vi "Dashboard Main.vi"() -> ()   [LabVIEW 2019]
uses:
  <vilib>/Rock Robotics/Network Tables/NT Read Numeric Array.vi
  <vilib>/Rock Robotics/Network Tables/NT Read Number.vi
  <vilib>/Rock Robotics/Network Tables/NT Read Boolean.vi
  <vilib>/Rock Robotics/Network Tables/NT Read String.vi
  <vilib>/Rock Robotics/Network Tables/NT Read Boolean Array.vi
  <vilib>/Rock Robotics/WPI/ThirdParty/JAS_Junk/TrajLib/Trajectory_Library.lvlib
panel:
  out "Camera Perf":string
  in  "Camera Settings":T1={"Frame Rate"=30, "Compression"=30, "Size"=1, "DB Camera Config"=FALSE} {"Frame Rate" scale=1.0..30.0; "Compression" scale=100.0..-1.0; "Size" items=["640x480", "320x240", "160x120"]}
  in  "TCP":refnum<k5>
  out "Robot IP":string
  in  "Dashboard Tab":T2(tab)
  out "MotorChart R":cluster{"Numeric":dbl, "Numeric":dbl}(graph)
  out "MotorChart L":cluster{"Numeric":dbl, "Numeric":dbl}(graph)
  out "MotorSliders R":cluster{"MotorSlide1":dbl, "MotorSlide2":dbl} {"MotorSlide2" scale=-1.0..1.0 scale format="%#_2e"; "MotorSlide1" scale=-1.0..1.0 scale format="%#_2e"}
  out "MotorSliders L":cluster{"MotorSlide1":dbl, "MotorSlide2":dbl} {"MotorSlide2" scale=-1.0..1.0 scale format="%#_2e"; "MotorSlide1" scale=-1.0..1.0 scale format="%#_2e"}
  out "JS1 Z":dbl(slide) scale=-1.0..1.0 scale format="%#_2e"
  out "JS1 Graph":cluster{"X":dbl, "Y":dbl}[](graph)
  out "JS1 Buttons":T3
  out "JS2 Z":dbl(slide) scale=-1.0..1.0 scale format="%#_2e"
  out "JS2 Graph":cluster{"X":dbl, "Y":dbl}[](graph)
  out "JS2 Buttons":T3
  out "Mode":T4(ring)=enum."Auto Disabled"
  in  "DB/String 9":string
  in  "DB/String 8":string
  in  "DB/String 7":string
  in  "DB/String 6":string
  in  "DB/String 5":string
  in  "DB/String 4":string
  in  "DB/String 3":string
  in  "DB/String 2":string
  in  "DB/String 1":string
  in  "DB/String 0":string
  in  "DB/Slider 0":dbl(slide) scale=0.0..5.0
  in  "DB/Slider 1":dbl(slide) scale=0.0..5.0
  in  "DB/Slider 2":dbl(slide) scale=0.0..5.0
  in  "DB/Slider 3":dbl(slide) scale=0.0..5.0
  out "DB/LED 3":bool
  out "DB/LED 2":bool
  out "DB/LED 1":bool
  out "DB/LED 0":bool
  in  "DB/Button 3":bool
  in  "DB/Button 2":bool
  in  "DB/Button 1":bool
  in  "DB/Button 0":bool caption="New Name"
  out "Gyro":dbl format="%10.1f"
  out "Gauge 2":dbl(knob) scale=-180.0..180.0
  out "Auto":bool
  out "R Err":dbl format="%9.2f"
  out "R Speed":dbl format="%10.1f"
  out "R Dmd":dbl format="%10.1f"
  out "L Err":dbl format="%9.2f"
  out "L Speed":dbl format="%10.1f"
  out "L Dmd":dbl format="%10.1f"
  out "NT Connection":bool
  in  "Select Auto":string(combo)="Select Autonomous ..."
  out "At Reference -":bool
  out "Ramsete Enabled -":bool
  out "Left Kp":dbl format="%13.3f"
  out "Left Ki":dbl format="%13.3f"
  out "Right Kp":dbl format="%13.3f"
  out "Right Ki":dbl format="%13.3f"
  out "Auto Tune Engaged":bool
  in  "Start Drive\nSpin Auto Tune":bool
  out "AutoTune\nRight Error":bool
  out "AutoTune\nLeft Error":bool
  out "AutoTune\nRight Done":bool
  out "AutoTune\nLeft Done":bool
  out "Test Name":string
  out "Test Step":string
  out "Test Step Time":dbl format="%16.1f"
  out "Left CO Offset":dbl format="%13.3f"
  out "Right CO Offset":dbl format="%13.3f"
  in  "Start Drive\nFwd Auto Tune":bool
  out "Drive Left":T5(graph)
  out "Drive Right":T5(graph)
  out "Ramsete Enabled":bool
  out "At Reference":bool
  out "Traj Error":T5(graph)
  out "Tree":string(tree)
  out "Camera Image":T6(plugin-control)
  out "Background":bool
  in  "Camera Name":string(combo)="No Camera Selection"
  # "HW"
  # "Joysticks"
  # "Drive Motors"
  # "Front"
  # "Right"
  # "Left"
  # "Back"
  # "Drive"
  # "Trajectory"
  # "Feet, Feet, Degrees/10"
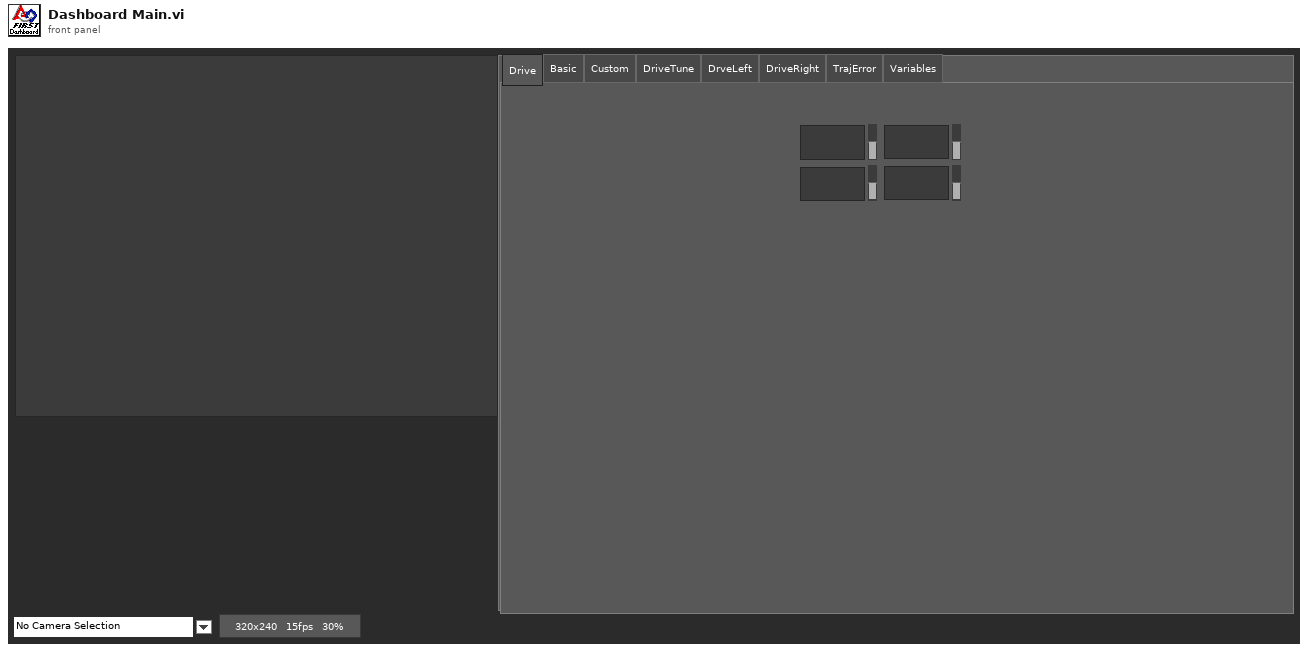
[diagram p1: front panel]
types:
  T1 = cluster{"Frame Rate":i32, "Compression":i32, "Size":u16, "DB Camera Config":bool}
  T2 = enum32{"Drive", "Basic", "Custom", "DriveTune", "DrveLeft", "DriveRight", "TrajError", "Variables"}
  T3 = cluster{bool, bool, bool, bool, bool, bool, bool, bool, bool, bool, bool, bool}
  T4 = enum8{"Tele-Op Disabled", "Tele-Op Enabled", "Auto Disabled", "Auto Enabled", "Test Disabled", "Test Enabled", "Disconnected", "No Code", "E-Stop"}
  T5 = cluster{"Numeric":dbl, "Numeric":dbl, "Numeric":dbl}
  T6 = typedef "IMAQ Image.ctl" = refnum<image>
  T7 = cluster{"Save Path":path, "Interval (s)":dbl, "Keep":i32}
  T8 = typedef "Image Type" = u32
  T9 = cluster{"Camera Image":refnum<vi>, "Dashboard Tab":refnum<vi>, "Background":refnum<vi>, "Tree":refnum<vi>, "Camera Settings":refnum<vi>, "Camera Name":refnum<vi>, "Camera Perf":refnum<vi>}
  T10 = cluster{"Shift":bool, "Ctrl":bool, "Alt":bool, "Cmd":bool, "Opt":bool}
  T11 = cluster{"Error Strings":string, "Disable Counts":cluster{u16, u16}, "Rail Faults":cluster{u16, u16, u16}, "Robot IP":string, "DB Mode":u8, "Event Info":cluster{"Name":string, "Type":u8, "Number":u16, "Replay":u8}}
  T12 = cluster{"Storage":cluster{"Disk Free":u64, "RAM Block":u32, "RAM free":u32}, "CPU Utilization":cluster{"CPU % ISR":sgl, "CPU % Time Crit":sgl, "CPU % Timed Str":sgl, "CPU % High":sgl, "CPU % Above":sgl, "CPU % Normal":sgl, "CPU % Low":sgl}, "CAN":cluster{"% Bus Utilization":sgl, "Bus Off Cnt":u32, "TX_FIFO Full Cnt":u32, "Receive Error Cnt":u8, "Transmit Error Cnt":u8}, "HID":cluster{"HID Outputs":u32, "Rumble Low":u16, "Rumble High":u16}[]}
  T13 = cluster{"Status bits":cluster{"Test Mode":bool, "Autonomous":bool, "Enabled":bool, "Code Start":bool, "Brownout":bool, "Reserved 2":bool, "Reserved 3":bool, "E-Stop":bool}, "Code Trace":cluster{"Disabled":bool, "TeleOp":bool, "Auto":bool, "Test":bool}, "Controller Type":enum16{"unknown", "cRIO", "roboRio"}, "Code?":enum16{"unknown", "noCode", "code"}, "Battery V":dbl}
  T14 = cluster{"Control Bits":cluster{"TestMode":bool, "Autonomous":bool, "Enabled":bool, "FMS Present":bool, bool, bool, bool, "E-Stop":bool}, "Team Station ":u8, "Countdown":sgl, "Joystick Values":cluster{"Axes":dbl[], "Buttons":bool[], "POVs":i16[]}[]}
  T15 = cluster{"Axes":dbl[], "Buttons":bool[], "POVs":i16[]}[]
  T16 = cluster{"Axes":dbl[], "Buttons":bool[], "POVs":i16[]}
  T17 = cluster{"Buttons[0]":bool, "Buttons[1]":bool, "Buttons[2]":bool, "Buttons[3]":bool, "Buttons[4]":bool, "Buttons[5]":bool, "Buttons[6]":bool, "Buttons[7]":bool, "Buttons[8]":bool, "Buttons[9]":bool, "Buttons[10]":bool, "Buttons[11]":bool}
  T18 = cluster{"Camera Name":string, "Camera File Name":string, "Saved DB Images Info":cluster{"Save Path":path, "Interval (s)":dbl, "Keep":i32}}
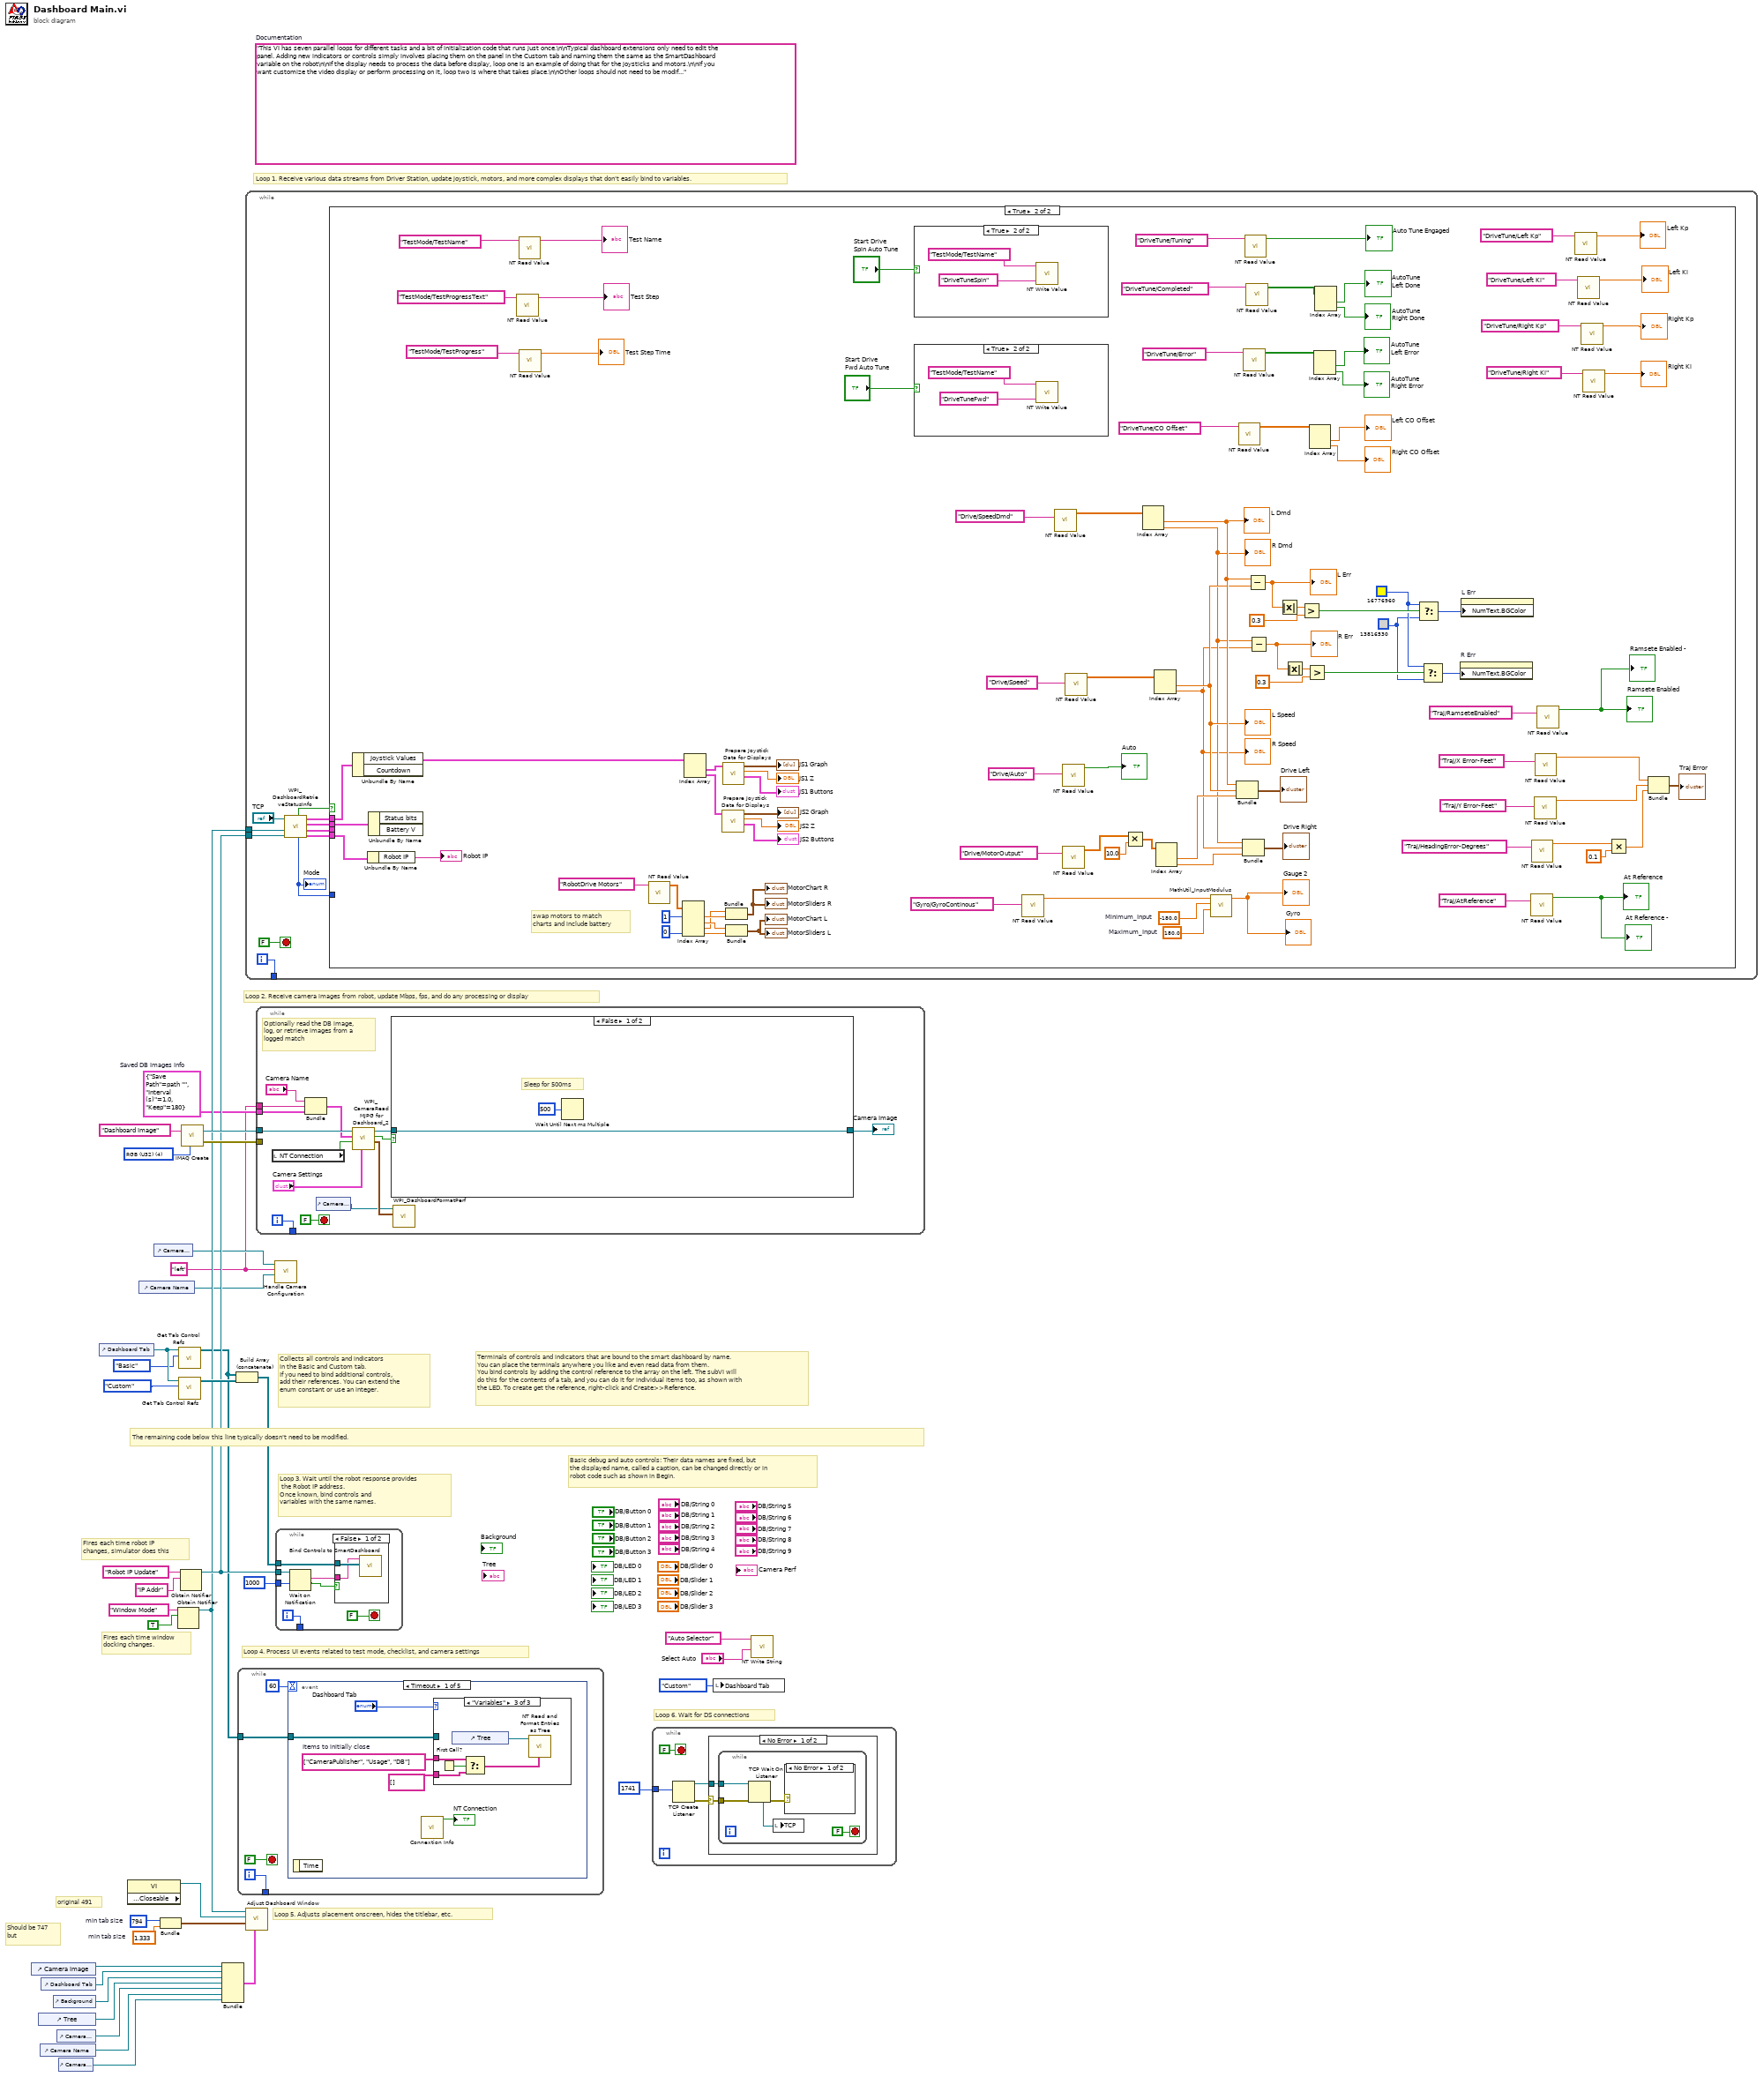
[diagram p0: block diagram]
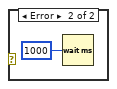
[diagram p2: hidden frame]
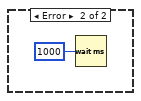
[diagram p3: hidden frame]
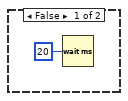
[diagram p4: hidden frame]
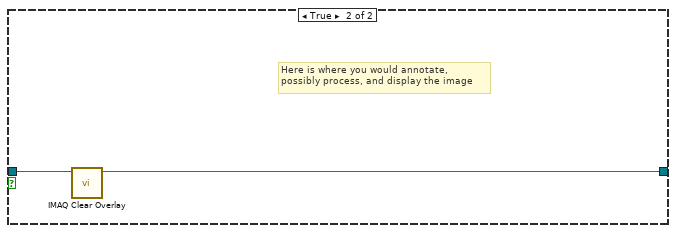
[diagram p8: hidden frame]
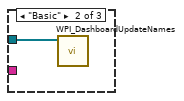
[diagram p10: hidden frame]
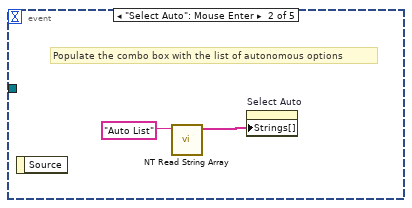
[diagram p11: hidden frame]
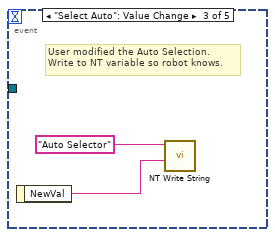
[diagram p12: hidden frame]
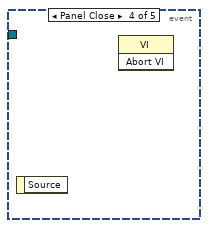
[diagram p13: hidden frame]
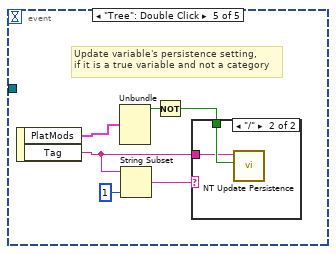
[diagram p14: hidden frame]
diagram:
  w2 = "left" ("Camera File Name")
  w3 = T7 {"Save Path"=path "", "Interval (s)"=1.0, "Keep"=180}  # Saved DB Images Info
  w22 = 794  # min tab size
  w21 = 1.333  # min tab size
  (unwired) "This VI has seven parallel loops for different tasks and a bit of initialization code that runs just once.\n\nTypical dashboard extensions only need to edit the panel. Adding new indicators or controls simply involves placing them on the panel in the Custom tab and naming them the same as the SmartDashboard variable on the robot\n\nIf the display needs to process the data before display, loop one is an example of doing that for the joysticks and motors.\n\nIf you want customize the video display or perform processing on it, loop two is where that takes place.\n\nOther loops should not need to be modified. They are pretty standard, and document the task they perform."  # Documentation
  w37 = T8 4 items=["Grayscale (U8)", "Grayscale (I16)", "Grayscale (SGL)", "Complex (CSG)", "RGB (U32)", "HSL (U32)", "RGB (U64)"] ("Image Type")
  # "Should be 747\nbut"
  # "original 491"
  # "Loop 6. Wait for DS connections"
  # "Basic debug and auto controls: Their data names are fixed, but\nthe displayed name, called a caption, can be changed directly or in\nrobot code such as shown in Begin."
  # "Fires each time robot IP\nchanges, simulator does this"
  # "Fires each time window\ndocking changes."
  # "Collects all controls and indicators\nin the Basic and Custom tab.\nIf you need to bind additional controls,\nadd their references. You can extend the\nenum constant or use an integer."
  # "The remaining code below this line typically doesn't need to be modified."
  # "Loop 4. Process UI events related to test mode, checklist, and camera settings"
  # "Terminals of controls and indicators that are bound to the smart dashboard by name.\nYou can place the terminals anywhere you like and even read data from them.\nYou bind controls by adding the control reference to the array on the left. The subVI will\ndo this for the contents of a tab, and you can do it for individual items too, as shown with\nthe LED. To create get the reference, right-click and Create>>Reference."
  # "Loop 3. Wait until the robot response provides\n the Robot IP address.\nOnce known, bind controls and\nvariables with the same names."
  # "Loop 5. Adjusts placement onscreen, hides the titlebar, etc."
  # "Loop 1. Receive various data streams from Driver Station, update joystick, motors, and more complex displays that don't easily bind to variables."
  # "Loop 2. Receive camera images from robot, update Mbps, fps, and do any processing or display"
  n1 = control-ref of="Camera Image"() -> (w24:refnum<vi>)
  n2 = control-ref of="Tree"() -> (w9:refnum<vi>)
  n3 = control-ref of="Camera Name"() -> (w7:refnum<vi>)
  n4 = control-ref of="Dashboard Tab"() -> (w23:refnum<vi>)
  n5 = control-ref of="Background"() -> (w19:refnum<vi>)
  n6 = control-ref of="Camera Settings"() -> (w8:refnum<vi>)
  n7 = control-ref of="Camera Perf"() -> (w6:refnum<vi>)
  n8 = control-ref of="Dashboard Tab"() -> (w27:refnum<vi>)
  n9 = property class="VI" props=["Front Panel.Closeable"]() -> (reference out=w28:refnum<vi>)  [unwired: 2 in, 2 out]
  n10 = control-ref of="Camera Name"() -> (w13:refnum<vi>)
  n11 = control-ref of="Camera Settings"() -> (w14:refnum<vi>)
  n12 = Bundle("min tab size"=w22, "min tab size"=w21) -> (w20:cluster{"min tab size":i32, "min tab size":dbl})  [unwired: 1 in]
  n13 = Obtain Notifier(name (unnamed)="Window Mode", notification data type=TRUE) -> (notifier out=w16:refnum<notifier>)  [unwired: 2 in, 2 out]
  n14 = call <vilib>:"Get Tab Control Refs.vi"("Page Index"=enum32{"Drive", "Basic", "Custom", "Variables"}."Basic" ("Dashboard Tab"), "TabControl in"=w27) -> ("ControlsOnPage"=w12:refnum<vi>[])  [unwired: 9 in]
  n15 = call <vilib>:"Get Tab Control Refs.vi"("Page Index"=enum32{"Drive", "Basic", "Custom", "Variables"}."Custom" ("Dashboard Tab"), "TabControl in"=w27) -> ("ControlsOnPage"=w26:refnum<vi>[])  [unwired: 9 in]
  n16 = Obtain Notifier(name (unnamed)="Robot IP Update", notification data type="IP Addr" ("name (unnamed)")) -> (notifier out=w17:refnum<notifier>)  [unwired: 2 in, 2 out]
  n17 = call "IMAQ Create"("Image Name"="Dashboard Image", "Image Type"=w37) -> ("New Image"=w35:T6, "error out"=w34:errorcluster)  [unwired: 2 in, 1 out]
  n18 = Bundle("Camera Image"=w24, "Dashboard Tab"=w23, "Background"=w19, "Tree"=w9, "Camera Settings"=w8, "Camera Name"=w7, "Camera Perf"=w6) -> (w18:T9)  [unwired: 1 in]
  n19 = Build Array (concatenate)(w12, w26) -> (w25:refnum<vi>[])
  n20 = while {
    tunnel: [w39] -> _
    tunnel: w12 -> [w38]
    i -> [w39]
    stop <- FALSE stop-if-true
    n21 = event shown="[0] Timeout" {
      selector: _ -> [_ _ _ _ _]
      dyn-events: _ -> [_ _ _ _ _]
      timeout: u32 60 ("milliseconds to wait") -> [_ _ _ _ _]
      tunnel: w38 -> [w44 _ _ _ _]
      event Timeout {
        w43 = string[] ["CameraPublisher", "Usage", "DB"]  # Items to initially close
        n22 = event-data() -> ()  [unwired: 1 in, 1 out]
        n23 = call <vilib>:"Connextion Info.vi"() -> ("Connected"=→"NT Connection":bool)  [unwired: 10 in, 1 out]
        n24 = case shown="\"Variables\"" "Dashboard Tab" {
          tunnel: w44 -> [_ w47 _]
          tunnel: w43 -> [_ _ w50]
          tunnel: string[] [] -> [_ _ w49]
          frame "Custom", Default {
          }
          frame "Basic" {
            n25 = call <vilib>:"WPI_DashboardUpdateNames.vi"("Controls on Tab"=w47) -> ()  [unwired: 11 in]
          }
          frame "Variables" {
            n26 = First Call?() -> (First Call?: T/F=w51:bool)
            n27 = control-ref of="Tree"() -> (w52:refnum<vi>)
            n28 = Select(t=w50, s=w51, f=w49) -> (s? t:f=w48:string[])
            n29 = call <vilib>:"NT Read and Format Entries as Tree.vi"("Tags to  Close"=w48, "Tree Refnum"=w52) -> ()  [unwired: 8 in, 2 out]
          }
        }
      }
      event "Select Auto": Mouse Enter {
        # "Populate the combo box with the list of autonomous options"
        n30 = event-data() -> ()  [unwired: 1 in, 1 out]
        n31 = call <vilib>:"NT Read String Array.vi"("Name"="Auto List") -> ("String Array"=w53:string[])  [unwired: 9 in, 1 out]
        n32 = property on="Select Auto" class="CmbBox"("Strings[]"=w53) -> ()  [unwired: 2 in, 2 out]
      }
      event "Select Auto": Value Change {
        # "User modified the Auto Selection.\nWrite to NT variable so robot knows."
        n33 = event-data() -> ("NewVal"=w55:string)  [unwired: 1 in]
        n34 = call <vilib>:"NT Write String.vi"("String"=w55, "Name"="Auto Selector") -> ()  [unwired: 9 in, 1 out]
      }
      event Panel Close {
        n35 = event-data() -> ()  [unwired: 1 in, 1 out]
        n36 = invoke class="VI" method="Abort VI"() -> ()  [unwired: 3 in, 3 out]
      }
      event "Tree": Double Click {
        # "Update variable's persistence setting,\nif it is a true variable and not a category"
        n37 = event-data() -> ("PlatMods"=w58:T10, "Tag"=w57:string)  [unwired: 1 in]
        n38 = Unbundle(w58) -> ("Shift"=w62:bool)  [unwired: 4 out]
        n39 = String Subset(string=w57, length (rest)=1 ("length (rest)")) -> (substring=w59:string)  [unwired: 1 in]
        n40 = Not(x=w62) -> (.not. x?=w61:bool)
        n41 = case shown="\"/\"" w59 {
          tunnel: w61 -> [_ w64]
          tunnel: w57 -> [_ w63]
          frame Default {
          }
          frame "/" {
            n42 = call <vilib>:"NT Update Persistence.vi"("Persistence"=w64, "Name"=w63) -> ()  [unwired: 9 in, 1 out]
          }
        }
      }
    }
  }
  n43 = while {
    tunnel: [w74] -> _
    tunnel: w17 -> [w68]
    tunnel: w16 -> [w65]
    i -> [w74]
    stop <- FALSE stop-if-true
    n44 = call <vilib>:"WPI_DashboardRetrieveStatusInfo.vi"("Binding Refnum"=w68, "Window Mode Notifier"=w65, "TCP Cnx"="TCP") -> ("Power and Errors"=w69:T11, "Robot Metrics"=w72:T12, "Status Info"=w73:T13, "Control Info"=w70:T14, "Robot Mode"=w67:T4, "Process?"=w71:bool)  [unwired: 3 in]
    "Mode" <- w67
    n45 = case shown="True" w71 {
      tunnel: w73 -> [_ w177]
      tunnel: w72 -> [_ _]
      tunnel: w70 -> [_ w176]
      tunnel: w69 -> [_ w175]
      tunnel: w67 -> [_ _]
      frame False {
        n46 = Wait (ms)(milliseconds to wait=u32 20) -> ()  [unwired: 1 out]
      }
      frame True {
        w115 = -180.0  # Minimum_Input
        w114 = 180.0  # Maximum_Input
        w119 = u32 13816530
        w120 = u32 16776960
        # "swap motors to match\ncharts and include battery"
        n47 = Unbundle By Name(w176) -> ("Joystick Values"=w166:T15)  [unwired: 1 out]
        n48 = Unbundle By Name(w175) -> ("Robot IP"=→"Robot IP":string)
        n49 = Unbundle By Name(w177) -> ()  [unwired: 2 out]
        n50 = call-poly <vilib>:"NT Read Value.vi"("Name"="TestMode/TestProgressText") -> ("String"=→"Test Step":string)  [unwired: 9 in, 1 out]
        n51 = call-poly <vilib>:"NT Read Value.vi"("Name"="TestMode/TestName") -> ("String"=→"Test Name":string)  [unwired: 9 in, 1 out]
        n52 = call-poly <vilib>:"NT Read Value.vi"("Name"="TestMode/TestProgress") -> ("Numeric"=→"Test Step Time":dbl)  [unwired: 9 in, 1 out]
        n53 = call-poly <vilib>:"NT Read Value.vi"("Name"="RobotDrive Motors") -> ("Numeric Array"=w156:dbl[])  [unwired: 9 in, 1 out]
        n54 = Index Array(array=w156, index #1=1, index #4=0) -> (element #1=w170:dbl, element #2=w171:dbl, element #3=w169:dbl, element #4=w174:dbl)  [unwired: 2 in]
        n55 = Index Array(array=w166) -> (element #1=w165:T16, element #2=w161:T16)  [unwired: 2 in]
        n56 = call "Prepare Joystick Data for Displays.vi"("Joystick Values"=w161) -> ("Buttons"=→"JS2 Buttons":T17, "Z Axis"=→"JS2 Z":dbl, "Cartesian Data"=→"JS2 Graph":cluster{"X axis":dbl, "X axis":dbl}[])  [unwired: 8 in]
        n57 = call "Prepare Joystick Data for Displays.vi"("Joystick Values"=w165) -> ("Buttons"=→"JS1 Buttons":T17, "Z Axis"=→"JS1 Z":dbl, "Cartesian Data"=→"JS1 Graph":cluster{"X axis":dbl, "X axis":dbl}[])  [unwired: 8 in]
        n58 = Bundle("Numeric"=w169, "Numeric"=w170) -> (→"MotorChart R" →"MotorSliders R":cluster{"Numeric":dbl, "Numeric":dbl})  [unwired: 1 in]
        n59 = Bundle("Numeric"=w171, "Numeric"=w174) -> (→"MotorChart L" →"MotorSliders L":cluster{"Numeric":dbl, "Numeric":dbl})  [unwired: 1 in]
        n60 = case shown="True" "Start Drive\nSpin Auto Tune" {
          frame False {
          }
          frame True {
            n61 = call-poly <vilib>:"NT Write Value.vi"("String"="DriveTuneSpin", "Name"="TestMode/TestName") -> ()  [unwired: 9 in, 1 out]
          }
        }
        n62 = case shown="True" "Start Drive\nFwd Auto Tune" {
          frame False {
          }
          frame True {
            n63 = call-poly <vilib>:"NT Write Value.vi"("String"="DriveTuneFwd", "Name"="TestMode/TestName") -> ()  [unwired: 9 in, 1 out]
          }
        }
        n64 = call-poly <vilib>:"NT Read Value.vi"("Name"="Gyro/GyroContinous") -> ("Numeric"=w113:dbl)  [unwired: 9 in, 1 out]
        n65 = call-poly <vilib>:"NT Read Value.vi"("Name"="Drive/SpeedDmd") -> ("Numeric Array"=w151:dbl[])  [unwired: 9 in, 1 out]
        n66 = call-poly <vilib>:"NT Read Value.vi"("Name"="Drive/Auto") -> ("Boolean"=→"Auto":bool)  [unwired: 9 in, 1 out]
        n67 = call-poly <vilib>:"NT Read Value.vi"("Name"="Drive/MotorOutput") -> ("Numeric Array"=w109:dbl[])  [unwired: 9 in, 1 out]
        n68 = call-poly <vilib>:"NT Read Value.vi"("Name"="Drive/Speed") -> ("Numeric Array"=w150:dbl[])  [unwired: 9 in, 1 out]
        n69 = Multiply(x=w109, y=10.0) -> (x*y=w108:dbl[])
        n70 = Index Array(array=w151) -> (element #1=w134:dbl, element #2=w132:dbl)  [unwired: 2 in]
        "L Dmd" <- w134
        "R Dmd" <- w132
        n71 = Index Array(array=w150) -> (element #1=w133:dbl, element #2=w131:dbl)  [unwired: 2 in]
        "L Speed" <- w133
        "R Speed" <- w131
        n72 = Index Array(array=w108) -> (element #1=w149:dbl, element #2=w148:dbl)  [unwired: 2 in]
        n73 = call <vilib>:"MathUtil_InputModulus.vi"("Maximum_Input"=w114, "Minimum_Input"=w115, "Input"=w113) -> ("modulus"=→"Gauge 2" →"Gyro":dbl)  [unwired: 8 in]
        n74 = Bundle("Numeric"=w134, "Numeric"=w133, w149) -> (→"Drive Left":cluster{"Numeric":dbl, "Numeric":dbl, dbl})  [unwired: 1 in]
        n75 = call-poly <vilib>:"NT Read Value.vi"("Name"="DriveTune/CO Offset") -> ("Numeric Array"=w80:dbl[])  [unwired: 9 in, 1 out]
        n76 = Bundle("Numeric"=w132, "Numeric"=w131, w148) -> (→"Drive Right":cluster{"Numeric":dbl, "Numeric":dbl, dbl})  [unwired: 1 in]
        n77 = call-poly <vilib>:"NT Read Value.vi"("Name"="DriveTune/Error") -> ("Boolean Array"=w95:bool[])  [unwired: 9 in, 1 out]
        n78 = call-poly <vilib>:"NT Read Value.vi"("Name"="DriveTune/Tuning") -> ("Boolean"=→"Auto Tune Engaged":bool)  [unwired: 9 in, 1 out]
        n79 = call-poly <vilib>:"NT Read Value.vi"("Name"="DriveTune/Completed") -> ("Boolean Array"=w94:bool[])  [unwired: 9 in, 1 out]
        n80 = Subtract(x=w134, y=w133) -> (x-y=w130:dbl)
        "L Err" <- w130
        n81 = Subtract(x=w132, y=w131) -> (x-y=w126:dbl)
        "R Err" <- w126
        n82 = Absolute Value(x=w130) -> (abs(x)=w129:dbl)
        n83 = Absolute Value(x=w126) -> (abs(x)=w127:dbl)
        n84 = Greater?(x=w129, y=0.3) -> (0:w124:bool)
        n85 = Greater?(x=w127, y=0.3) -> (0:w122:bool)
        n86 = Index Array(array=w80) -> (element #1=→"Left CO Offset":dbl, element #2=→"Right CO Offset":dbl)  [unwired: 2 in]
        n87 = Index Array(array=w95) -> (element #1=→"AutoTune\nLeft Error":bool, element #2=→"AutoTune\nRight Error":bool)  [unwired: 2 in]
        n88 = Index Array(array=w94) -> (element #1=→"AutoTune\nLeft Done":bool, element #2=→"AutoTune\nRight Done":bool)  [unwired: 2 in]
        n89 = Select(t=w120, s=w124, f=w119) -> (s? t:f=w123:u32)
        n90 = Select(t=w120, s=w122, f=w119) -> (s? t:f=w121:u32)
        n91 = property on="R Err" class="DigNum (strict)"("NumText.BGColor"=w121) -> ()  [unwired: 2 in, 2 out]
        n92 = property on="L Err" class="DigNum (strict)"("NumText.BGColor"=w123) -> ()  [unwired: 2 in, 2 out]
        n93 = call-poly <vilib>:"NT Read Value.vi"("Name"="Traj/AtReference") -> ("Boolean"=→"At Reference" →"At Reference -":bool)  [unwired: 9 in, 1 out]
        n94 = call-poly <vilib>:"NT Read Value.vi"("Name"="Traj/HeadingError-Degrees") -> ("Numeric"=w138:dbl)  [unwired: 9 in, 1 out]
        n95 = call-poly <vilib>:"NT Read Value.vi"("Name"="Traj/Y Error-Feet") -> ("Numeric"=w141:dbl)  [unwired: 9 in, 1 out]
        n96 = call-poly <vilib>:"NT Read Value.vi"("Name"="Traj/X Error-Feet") -> ("Numeric"=w142:dbl)  [unwired: 9 in, 1 out]
        n97 = call-poly <vilib>:"NT Read Value.vi"("Name"="Traj/RamseteEnabled") -> ("Boolean"=→"Ramsete Enabled" →"Ramsete Enabled -":bool)  [unwired: 9 in, 1 out]
        n98 = call-poly <vilib>:"NT Read Value.vi"("Name"="DriveTune/Left Kp") -> ("Numeric"=→"Left Kp":dbl)  [unwired: 9 in, 1 out]
        n99 = call-poly <vilib>:"NT Read Value.vi"("Name"="DriveTune/Left Ki") -> ("Numeric"=→"Left Ki":dbl)  [unwired: 9 in, 1 out]
        n100 = call-poly <vilib>:"NT Read Value.vi"("Name"="DriveTune/Right Kp") -> ("Numeric"=→"Right Kp":dbl)  [unwired: 9 in, 1 out]
        n101 = call-poly <vilib>:"NT Read Value.vi"("Name"="DriveTune/Right Ki") -> ("Numeric"=→"Right Ki":dbl)  [unwired: 9 in, 1 out]
        n102 = Multiply(x=w138, y=0.1) -> (x*y=w137:dbl)
        n103 = Bundle("Numeric"=w142, "Numeric"=w141, w137) -> (→"Traj Error":cluster{"Numeric":dbl, "Numeric":dbl, dbl})  [unwired: 1 in]
      }
    }
  }
  n104 = call "Adjust Dashboard Window.vi"("Sizing Refnums"=w18, "Size Constraints"=w20, "VI"=w28, "WIn Mode"=w16) -> ()  [unwired: 8 in]
  n105 = while {
    tunnel: w35 -> [w193]
    tunnel: w34 -> [_]
    tunnel: [w194] -> _
    tunnel: w3 -> [w187]
    tunnel: w2 -> [w184]
    i -> [w194]
    stop <- FALSE stop-if-true
    # "Optionally read the DB image,\nlog, or retrieve images from a\nlogged match"
    n106 = local read "NT Connection"() -> (w188:bool)
    n107 = Bundle("Camera Name"="Camera Name", "Camera File Name"=w184, "Saved DB Images Info"=w187) -> (w186:T18)  [unwired: 1 in]
    n108 = control-ref of="Camera Perf"() -> (w182:refnum<vi>)
    n109 = call <vilib>:"WPI_CameraRead MJPG for Dashboard_2.vi"("Camera Settings"="Camera Settings", "NT Connection"=w188, "Capture Info"=w186, "Image in"=w193) -> ("perf info"=w183:cluster{"Bandwidth (Mbps)":dbl, "fps":dbl}, "Active"=w191:bool, "Image\\ out"=w192:T6)  [unwired: 5 in]
    n110 = case shown="False" w191 {
      tunnel: w192 -> [w196 w199]
      tunnel: [w196 w198] -> w189
      frame False {
        # "Sleep for 500ms"
        n111 = Wait Until Next ms Multiple(millisecond multiple=u32 500) -> ()  [unwired: 1 out]
      }
      frame True {
        # "Here is where you would annotate,\npossibly process, and display the image"
        n112 = call "IMAQ Clear Overlay"("Image"=w199) -> ("Image Out"=w198:T6)  [unwired: 2 in, 8 out]
      }
    }
    "Camera Image" <- w189
    n113 = call <vilib>:"WPI_DashboardFormatPerf.vi"("Performance"=w183, "String in"=w182) -> ()  [unwired: 10 in]
  }
  n114 = call "Handle Camera Configuration.vi"("CameraNameRef"=w13, "Display Name"=w2, "ClusterRef"=w14) -> ()  [unwired: 9 in]
  n115 = while {
    tunnel: w25 -> [w206]
    tunnel: w17 -> [w204]
    tunnel: [w202] -> _
    tunnel: u32 1000 ("milliseconds to wait") -> [w201]
    i -> [w202]
    stop <- FALSE stop-if-true
    n116 = Wait on Notification(notifier=w204, timeout in ms (-1)=w201) -> (notification=w203:string, timed out?=w200:bool)  [unwired: 2 in, 2 out]
    n117 = case shown="False" w200 {
      tunnel: w206 -> [w208 _]
      tunnel: w203 -> [w207 _]
      frame False {
        n118 = call <vilib>:"Bind Controls to SmartDashboard.vi"("Bound Control Refs"=w208, "Server IP Address"=w207) -> ()  [unwired: 10 in]
      }
      frame True {
      }
    }
  }
  n119 = while {
    tunnel: u16 1741 ("timeout ms (25000)") -> [w210]
    stop <- FALSE stop-if-true
    n120 = TCP Create Listener(10:w210) -> (0:w209:errorcluster, 3:w211:refnum<k5>)  [unwired: 4 in, 1 out]
    n121 = case shown="No Error" w209 {
      selector: w209 -> [w213 _]
      tunnel: w211 -> [w214 _]
      frame No Error {
        n122 = while {
          tunnel: w214 -> [w217]
          tunnel: w213 -> [w216]
          stop <- FALSE stop-if-true
          n123 = TCP Wait On Listener(8:w216, 11:w217) -> (0:w218:errorcluster, 4:w219:refnum<k5>)  [unwired: 2 in, 3 out]
          n124 = local write "TCP"(w219) -> ()
          n125 = case shown="No Error" w218 {
            frame No Error {
            }
            frame Error {
              n126 = Wait (ms)(milliseconds to wait=u32 1000) -> ()  [unwired: 1 out]
            }
          }
        }
      }
      frame Error {
        n127 = Wait (ms)(milliseconds to wait=u32 1000) -> ()  [unwired: 1 out]
      }
    }
  }
  n128 = local write "Dashboard Tab"(T2."Custom" ("Dashboard Tab")) -> ()
  n129 = call <vilib>:"NT Write String.vi"("String"="Select Auto", "Name"="Auto Selector") -> ()  [unwired: 9 in, 1 out]
